vi "Update Tip Coordinates.vi"(4 "Scale Coorection Factor":cluster{"Kx":dbl, "Ky":dbl, "Kz":dbl}={"Kx"=1.0, "Ky"=1.0, "Kz"=1.0}, 5 "Angles":cluster{"phi [rad]":dbl, "theta [rad]":dbl}, 6 "Transformation Matrix":T2, 7 "Initial Manipulator Coordinates":T1, 10 "Initial Tip Coordinates":T1, 11 "Current Manipulator Coordinates":T1) -> (2 "Current Coordinates":T1)   [LabVIEW 2012, in "Targeting Unit.lvlib"]
uses:
  Targeting Unit.lvlib
  <vilib>/Analysis/Matrix/Datatypes/RealMatrix.ctl
  <vilib>/Analysis/Matrix/NI_Matrix.lvlib
panel:
  # "X entering (1) or exiting tip (-1)"
  # "Flip (Yes -1 No 1)"
  # "Insertion step coefficient"
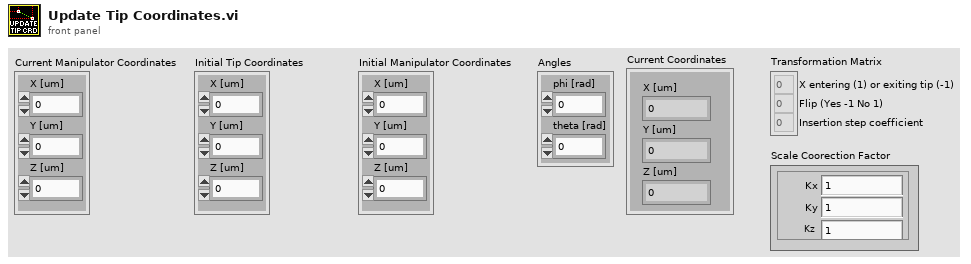
[diagram p1: front panel]
types:
  T1 = cluster{"X [um]":dbl, "Y [um]":dbl, "Z [um]":dbl}
  T2 = typedef "NI_Matrix.lvlib/RealMatrix.ctl" = dbl[][]
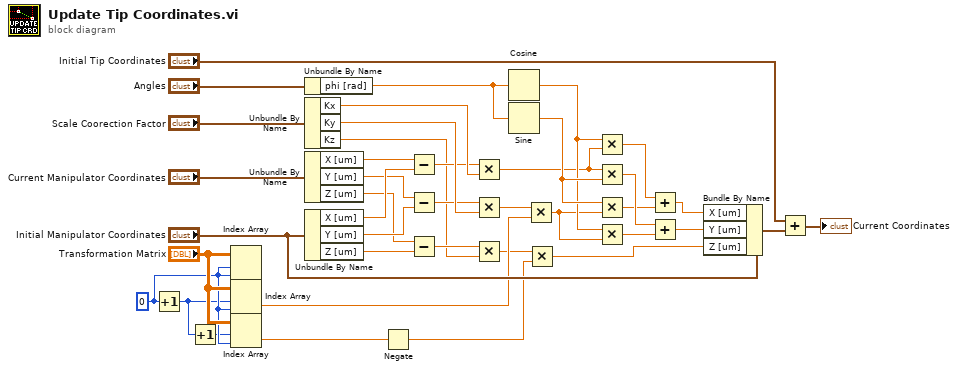
[diagram p0: block diagram]
diagram:
  w24 = 0 ("index (col)")
  n1 = Increment(x=w24) -> (x+1=w22:i32)
  n2 = Increment(x=w22) -> (x+1=w23:i32)
  n3 = Index Array(array="Transformation Matrix", index (row)=w24, index (col)=w24) -> ()  [unwired: 1 out]
  n4 = Index Array(array="Transformation Matrix", index (row)=w22, index (col)=w24) -> (element=w16:dbl)
  n5 = Index Array(array="Transformation Matrix", index (row)=w23, index (col)=w24) -> (element=w25:dbl)
  n6 = Unbundle By Name("Angles") -> ("phi [rad]"=w33:dbl)
  n7 = Unbundle By Name("Scale Coorection Factor") -> ("Kx"=w12:dbl, "Ky"=w11:dbl, "Kz"=w1:dbl)
  n8 = Unbundle By Name("Current Manipulator Coordinates") -> ("X [um]"=w40:dbl, "Y [um]"=w38:dbl, "Z [um]"=w35:dbl)
  n9 = Unbundle By Name("Initial Manipulator Coordinates") -> ("X [um]"=w39:dbl, "Y [um]"=w37:dbl, "Z [um]"=w36:dbl)
  n10 = Negate(x=w25) -> (-x=w15:dbl)
  n11 = Subtract(x=w40, y=w39) -> (x-y=w7:dbl)
  n12 = Subtract(x=w38, y=w37) -> (x-y=w8:dbl)
  n13 = Subtract(x=w35, y=w36) -> (x-y=w4:dbl)
  n14 = Multiply(x=w7, y=w12) -> (x*y=w6:dbl)
  n15 = Multiply(x=w8, y=w11) -> (x*y=w5:dbl)
  n16 = Multiply(x=w4, y=w1) -> (x*y=w3:dbl)
  n17 = Cosine(x=w33) -> (cos(x)=w29:dbl)
  n18 = Sine(x=w33) -> (sin(x)=w30:dbl)
  n19 = Multiply ("Multiply.vi")(x=w5, y=w16) -> (x*y=w17:dbl)
  n20 = Multiply ("Multiply.vi")(x=w3, y=w15) -> (x*y=w31:dbl)
  n21 = Multiply(x=w29, y=w6) -> (x*y=w20:dbl)
  n22 = Multiply(x=w6, y=w30) -> (x*y=w21:dbl)
  n23 = Multiply(x=w30, y=w17) -> (x*y=w19:dbl)
  n24 = Multiply(x=w29, y=w17) -> (x*y=w18:dbl)
  n25 = Add(x=w20, y=w19) -> (x+y=w10:dbl)
  n26 = Add(x=w21, y=w18) -> (x+y=w9:dbl)
  n27 = Bundle By Name(cluster="Initial Manipulator Coordinates", "X [um]"=w10, "Y [um]"=w9, "Z [um]"=w31) -> (w28:T1)
  n28 = Add(x="Initial Tip Coordinates", y=w28) -> (x+y=→"Current Coordinates":T1)
